vi "Send UDP Packet.vi"(6 "connection info in":T1, 8 "error in (no error)":errorcluster, 11 "Assert Message in":T3) -> (0 "error out":errorcluster)   [LabVIEW 2016, in "Assert API Components.lvlib" / "Log Assert Core.lvlib"]
doc: "Sends the message back over the UDP port to the main display with the relevant data"
uses:
  Log Assert Core.lvlib
  Message Data.ctl
  Failure Actions.ctl
  VI References.ctl
  <vilib>/NI/STM/TCP/TCP Connection Info.ctl
  <vilib>/NI/STM/SubVIs/MetaDataElement.ctl
  <vilib>/NI/STM/TCP/Write Message (TCP).vi
  <vilib>/NI/STM/NI STM.lvlib
  Assert API Components.lvlib
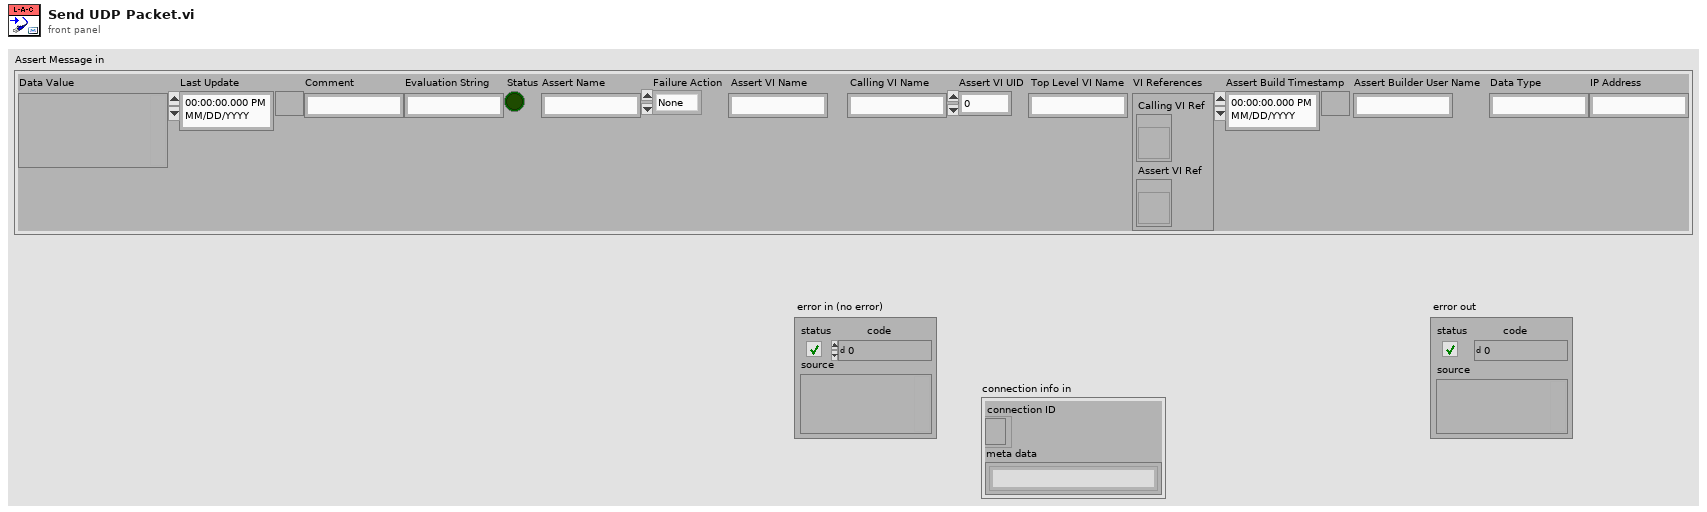
[diagram p1: front panel]
types:
  T1 = typedef "NI STM.lvlib/TCP Connection Info.ctl" = cluster{"connection ID":refnum<k5>, "meta data":T2[]}
  T2 = typedef "NI STM.lvlib/MetaDataElement.ctl" = string
  T3 = typedef "Assert API Components.lvlib/Message Data.ctl" = cluster{"Data Value":variant, "Last Update":timestamp, "Comment":string, "Evaluation String":string, "Status":bool, "Assert Name":string, "Failure Action":T4, "Assert VI Name":string, "Calling VI Name":string, "Assert VI UID":i32, "Top Level VI Name":string, "VI References":T5, "Assert Build Timestamp":timestamp, "Assert Builder User Name":string, "Data Type":string, "IP Address":string}
  T4 = typedef "Assert API Components.lvlib/Failure Actions.ctl" = enum16{"None", "Log To File", "Pause Execution", "Abort Execution"}
  T5 = typedef "Assert API Components.lvlib/VI References.ctl" = cluster{"Calling VI Ref":refnum<vi>, "Assert VI Ref":refnum<vi>}
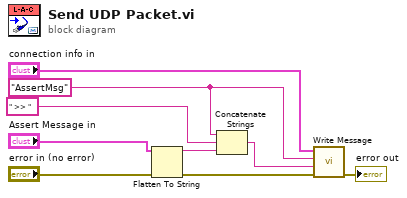
[diagram p0: block diagram]
diagram:
  w4 = "AssertMsg" ("name")
  n1 = Flatten To String(anything="Assert Message in", error in (no error)="error in (no error)") -> (data string=w2:string, error out=w8:errorcluster)  [unwired: 2 in, 1 out]
  n2 = Concatenate Strings(w4, " >> " ("string"), w2) -> (w1:string)
  n3 = call-poly <vilib>:"Write Message.vi"("error in"=w8, "data"=w1, "name"=w4, "connection info in"="connection info in") -> ("error out"=→"error out":errorcluster)  [unwired: 6 in, 1 out]
